vi "Table Select.vi"() -> ()   [LabVIEW 2019]
uses:
  <vilib>/Utility/miscctls.llb/LVPositionTypeDef.ctl
  <vilib>/Utility/miscctls.llb/LVPointTypeDef.ctl
  LLB/Message/Ctrl/MsgDataInput.ctl
  LLB/Message/Ctrl/MsgPageSelect.ctl
  LLB/Message/Ctrl/LogType.ctl
  LLB/Message/MsgShowAndLog.lvlib
  LLB/Commonly VI.lvlib
panel:
  in  "Tab Control":refnum<vi>
  in  "Variant":variant
  out "Class ID":u32
  out "Class Name":string
  out "OldVal":variant
  out "NewVal":variant
  out "size(s)":i32
  in  "Tab Control":enum32{"Page 1", "Page 2"}(tab)
  in  "Save":bool
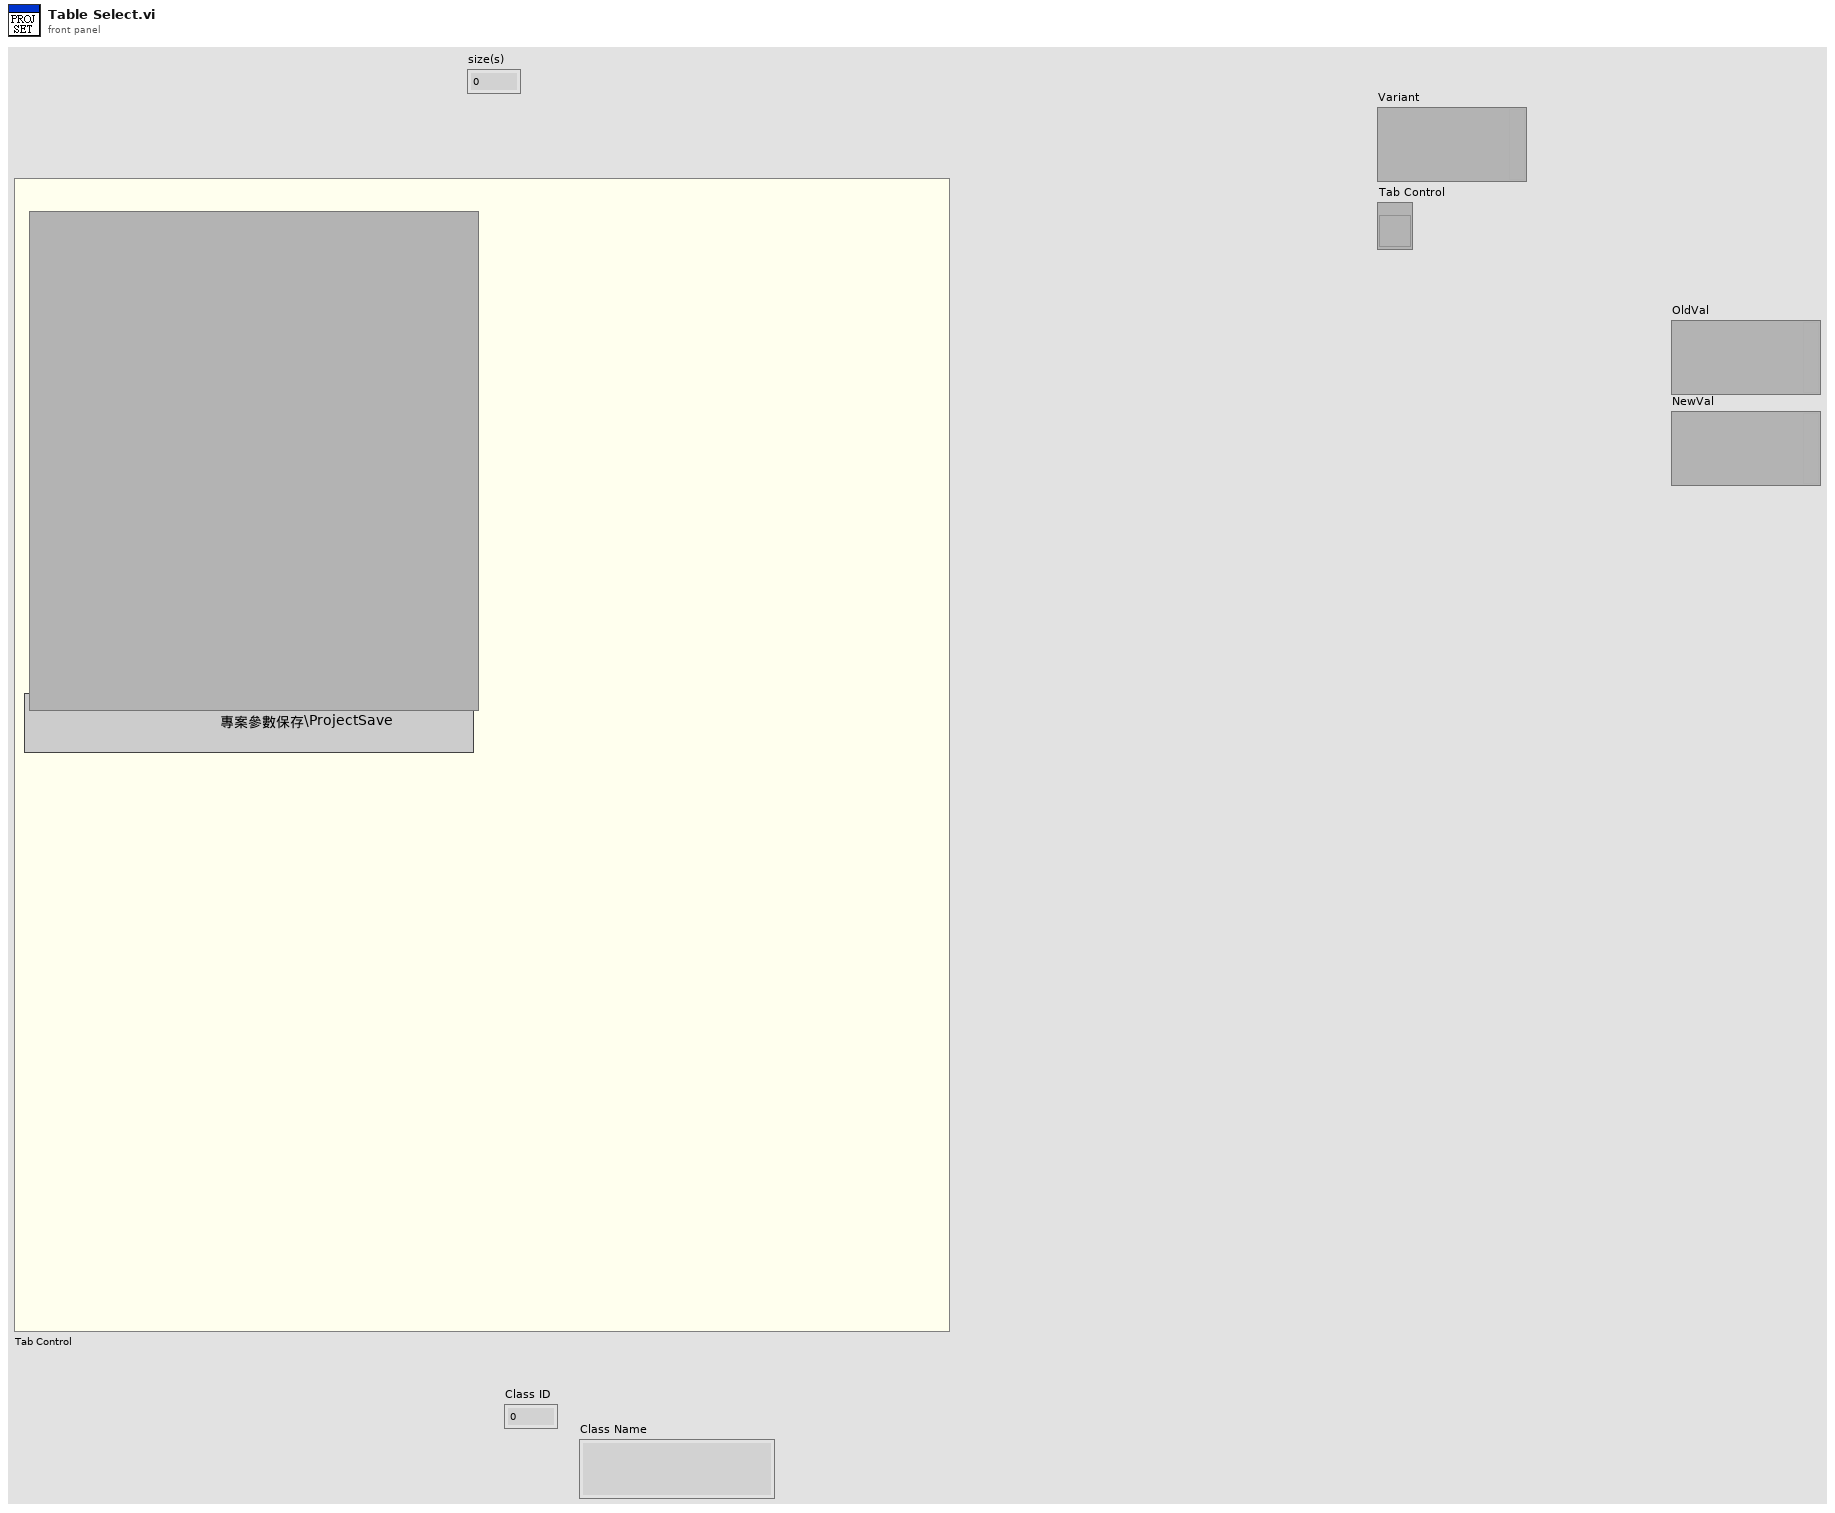
[diagram p1: front panel]
types:
  T1 = typedef "LVPositionTypeDef.ctl" = cluster{"Left":i32, "Top":i32}
  T2 = typedef "LVPointTypeDef.ctl" = cluster{"Horizontal":i16, "Vertical":i16}
  T3 = typedef "MsgDataInput.ctl" = cluster{"MsgPageSelect":T4, "LogType":T5, "Msg":string, "Time":string}
  T4 = typedef "MsgShowAndLog.lvlib/MsgPageSelect.ctl" = enum16{"System", "Comm", "IO", "Action", "Alarm"}
  T5 = typedef "MsgShowAndLog.lvlib/LogType.ctl" = enum16{"Auto", "Manual", "Handshake", "Error"}
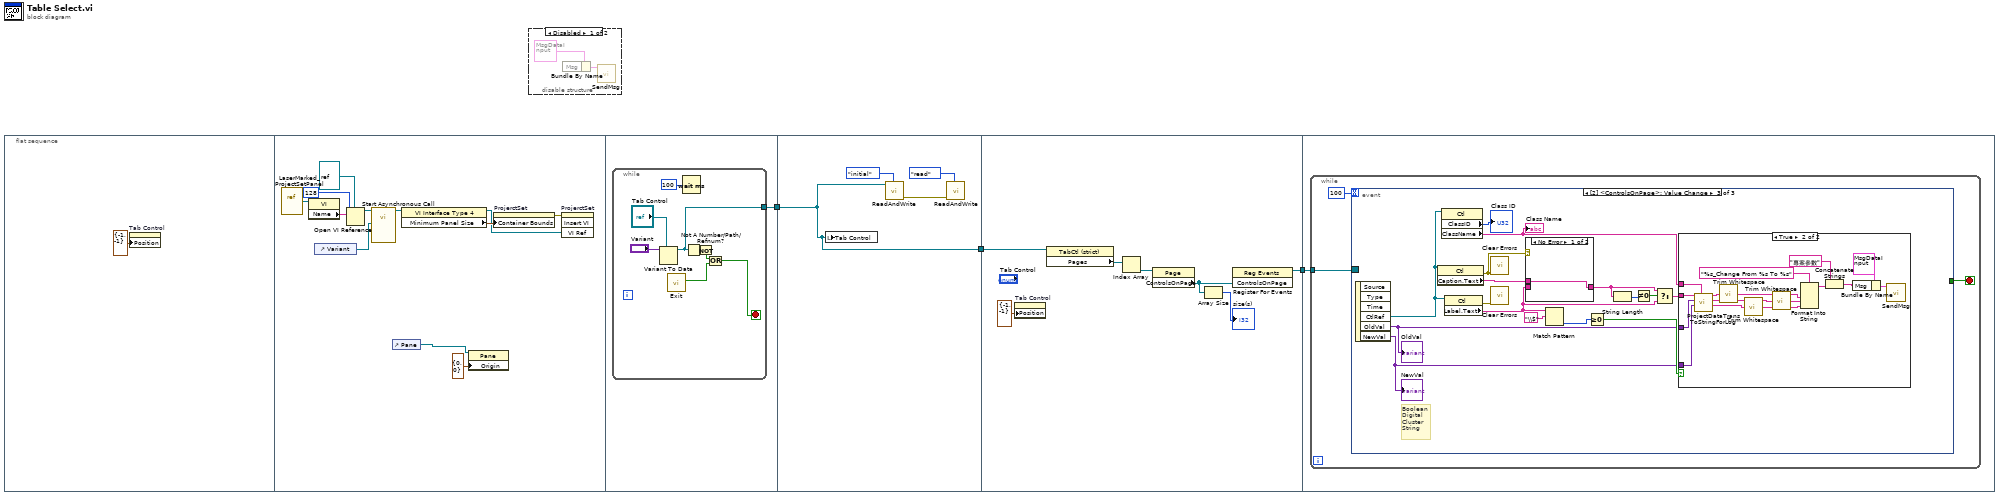
[diagram p0: block diagram]
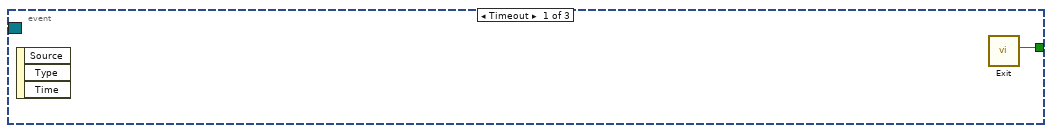
[diagram p3: hidden frame]
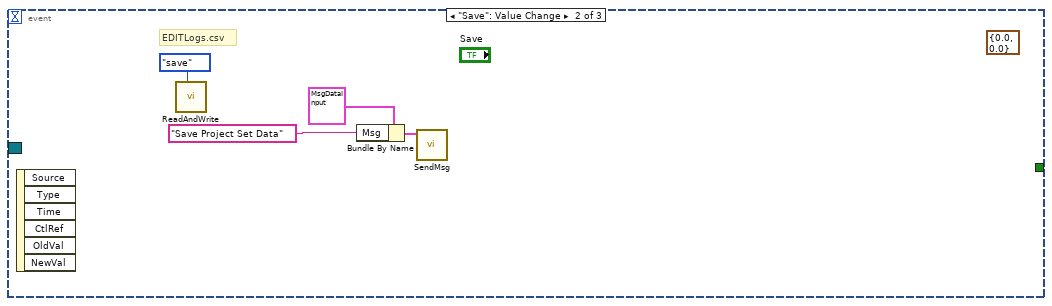
[diagram p4: hidden frame]
diagram:
  n1 = flat-sequence {
    tunnel: [w17] -> w2
    tunnel: w2 -> [w26]
    tunnel: [w26] -> w1
    tunnel: [w35] -> w3
    tunnel: w1 -> [w30]
    tunnel: w3 -> [w37]
    frame #0 {
      n2 = property on="Tab Control" class="TabCtl (strict)"("Position"=T1 {"Left"=-1, "Top"=-1}) -> ()  [unwired: 2 in, 2 out]
    }
    frame #1 {
      n3 = vi-ref "LaserMarked_ProjectSetPanel.vi"() -> (w16:refnum<vi>)
      n4 = property class="VI"(reference=w16) -> ("Name"=w15:string)  [unwired: 1 in, 2 out]
      n5 = control-ref of="Variant"() -> (w8:refnum<vi>)
      n6 = Open VI Reference(type specifier VI Refnum (for type only)=refnum<vi> refnum, vi path=w15, options=128) -> (vi reference=w10:refnum<vi>)  [unwired: 3 in, 1 out]
      n7 = call-by-ref "Start Asynchronous Call"(reference=w10, "SetPanelRef"=w8) -> (reference out=w9:refnum<vi>)  [unwired: 12 in, 1 out]
      n8 = control-ref of="Pane"() -> (w5:refnum<vi>)
      n9 = property class="VI Interface Type 4"(reference=w9) -> (reference out=w12:refnum<vi>, "Minimum Panel Size"=w13:T2)  [unwired: 1 in, 1 out]
      n10 = property class="Pane"(reference=w5, "Origin"=T2 {"Horizontal"=0, "Vertical"=0}) -> ()  [unwired: 1 in, 2 out]
      n11 = property on="ProjerctSet" class="SubPnl"("Container Bounds"=w13) -> (error out=w11:errorcluster)  [unwired: 2 in, 1 out]
      n12 = invoke on="ProjerctSet" class="SubPnl" method="Insert VI"(error in=w11, "VI Ref"=w12) -> ()  [unwired: 2 in, 4 out]
    }
    frame #2 {
      n13 = while {
        tunnel: [w22] -> w17
        stop <- w20 stop-if-true
        n14 = Variant To Data(type="Tab Control", Variant="Variant") -> (data=w22:refnum<vi>)  [unwired: 1 in, 1 out]
        n15 = call "Exit.vi"() -> ("ExitOut"=w19:bool)  [unwired: 11 in]
        n16 = Wait (ms)(milliseconds to wait=u32 100) -> ()  [unwired: 1 out]
        n17 = Not A Number/Path/Refnum?(number/path/refnum=w22) -> (NaN/Path/Refnum?=w21:bool)
        n18 = Not(x=w21) -> (.not. x?=w18:bool)
        n19 = Or(x=w18, y=w19) -> (x .or. y?=w20:bool)
      }
    }
    frame #3 {
      n20 = local write "Tab Control"(w26) -> ()
      n21 = call "ReadAndWrite.vi"("Enum"=enum16{"initial", "save", "read"}."initial", "Tab Control"=w26) -> ("error out"=w27:errorcluster)  [unwired: 9 in]
      n22 = call "ReadAndWrite.vi"("Enum"=enum16{"initial", "save", "read"}."read", "error in"=w27) -> ()  [unwired: 9 in, 1 out]
    }
    frame #4 {
      n23 = property on="Tab Control" class="TabCtl (strict)"("Position"=T1 {"Left"=-1, "Top"=-1}) -> ()  [unwired: 2 in, 2 out]
      n24 = property class="TabCtl (strict)"(reference=w30) -> ("Pages"=w33:refnum<vi>[])  [unwired: 1 in, 2 out]
      n25 = Index Array(array=w33) -> (element=w32:refnum<vi>)  [unwired: 1 in]
      n26 = property class="Page"(reference=w32) -> ("ControlsOnPage"=w31:refnum<vi>[])  [unwired: 1 in, 2 out]
      n27 = Array Size(array=w31) -> (size(s)=→"size(s)":i32)
      n28 = register-events(w31) -> (reference out=w35:refnum<event-registration>)  [unwired: 2 in, 1 out]
    }
    frame #5 {
      n29 = while {
        tunnel: w37 -> [w38]
        stop <- w39 stop-if-true
        n30 = event shown="[2] <ControlsOnPage>: Value Change" {
          selector: w38 -> [_ _ _]
          dyn-events: _ -> [_ _ _]
          timeout: 100 -> [_ _ _]
          tunnel: [w41 _ _] -> w39
          event Timeout {
            n31 = event-data() -> ()  [unwired: 1 in, 3 out]
            n32 = call "Exit.vi"() -> ("ExitOut"=w41:bool)  [unwired: 11 in]
          }
          event "Save": Value Change {
            (unwired) cluster{"Max":dbl, "Min":dbl} {"Max"=0.0, "Min"=0.0} ("BinRange")
            # "EDITLogs.csv"
            n33 = event-data() -> ()  [unwired: 1 in, 6 out]
            n34 = call "ReadAndWrite.vi"("Enum"=enum16{"initial", "save", "read"}."save") -> ()  [unwired: 10 in, 1 out]
            n35 = Bundle By Name(cluster=T3 {"MsgPageSelect"=enum."System", "LogType"=enum."Manual", "Msg"="刪除專案 KKI", "Time"=""} ("DataIn"), "Msg"="Save Project Set Data") -> (w44:T3)
            n36 = call "SendMsg.vi"("DataIn"=w44) -> ()  [unwired: 10 in, 1 out]
          }
          event Value Change {
            # "Boolean\nDigital\nCluster\nString"
            n37 = event-data() -> ("CtlRef"=w51:refnum<vi>, "OldVal"=w56:variant, "NewVal"=w57:variant)  [unwired: 1 in, 3 out]
            "OldVal" <- w56
            "NewVal" <- w57
            n38 = property class="Ctl"(reference=w51) -> (error out=w49:errorcluster, "Caption.Text"=w47:string)  [unwired: 1 in, 1 out]
            n39 = property class="Ctl"(reference=w51) -> ("ClassID"=→"Class ID":u32, "ClassName"=w55:string)  [unwired: 1 in, 2 out]
            "Class Name" <- w55
            n40 = property class="Ctl"(reference=w51) -> (error out=w50:errorcluster, "Label.Text"=w46:string)  [unwired: 1 in, 1 out]
            n41 = call <vilib>:"Clear Errors.vi"("error in (no error)"=w49) -> ()  [unwired: 5 in, 2 out]
            n42 = call <vilib>:"Clear Errors.vi"("error in (no error)"=w50) -> ()  [unwired: 5 in, 2 out]
            n43 = case shown="No Error" w49 {
              tunnel: [w62 w63] -> w48
              tunnel: w47 -> [w62 _]
              tunnel: w46 -> [_ w63]
              frame No Error {
              }
              frame Error {
              }
            }
            n44 = Match Pattern(string=w46, regular expression="\\$") -> (offset past match=w59:i32)  [unwired: 1 in, 3 out]
            n45 = Greater Or Equal To 0?(x=w59) -> (x >= 0?=w58:bool)
            n46 = String Length(string=w48) -> (length=w54:i32)
            n47 = Not Equal To 0?(x=w54) -> (x != 0?=w53:bool)
            n48 = Select(t=w48, s=w53, f=w46) -> (s? t:f=w52:string)
            n49 = case shown="True" w58 {
              tunnel: w56 -> [_ w76]
              tunnel: w57 -> [_ w75]
              tunnel: w52 -> [_ w67]
              tunnel: w55 -> [_ w66]
              frame False {
              }
              frame True {
                n50 = call "ProjectDataTransToStringForLog.vi"("Class Name"=w66, "NewVal"=w75, "OldVal"=w76, "Label.Text"=w67) -> ("NewData"=w73:string, "OldData"=w74:string, "DataName"=w77:string)  [unwired: 5 in]
                n51 = call <vilib>:"Trim Whitespace.vi"("string"=w77) -> ("trimmed string"=w78:string)  [unwired: 1 in]
                n52 = call <vilib>:"Trim Whitespace.vi"("string"=w73) -> ("trimmed string"=w71:string)  [unwired: 1 in]
                n53 = call <vilib>:"Trim Whitespace.vi"("string"=w74) -> ("trimmed string"=w72:string)  [unwired: 1 in]
                n54 = Format Into String(format string="%s_Change From %s To %s", w78, w72, w71) -> (resulting string=w68:string)  [unwired: 2 in, 1 out]
                n55 = Concatenate Strings("專案參數" ("string"), w68) -> (w65:string)
                n56 = Bundle By Name(cluster=T3 {"MsgPageSelect"=enum."System", "LogType"=enum."Manual", "Msg"="刪除專案 KKI", "Time"=""} ("DataIn"), "Msg"=w65) -> (w69:T3)
                n57 = call "SendMsg.vi"("DataIn"=w69) -> ()  [unwired: 10 in, 1 out]
              }
            }
          }
        }
      }
    }
  }
  n58 = disable-structure shown="Disabled" {
    frame Disabled {
      n59 = Bundle By Name(cluster=T3 {"MsgPageSelect"=enum."System", "LogType"=enum."Manual", "Msg"="刪除專案 KKI", "Time"=""} ("DataIn")) -> (w81:T3)  [unwired: 1 in]
      n60 = call "SendMsg.vi"("DataIn"=w81) -> ()  [unwired: 10 in, 1 out]
    }
    frame Enabled {
    }
  }
